vi "createInboundChannel.vi"(8 "error in (no error)":errorcluster, 11 "Connection.TCP in":refnum<class "Connection.TCP.lvclass">) -> (0 "error out":errorcluster, 2 "Authorization":T1, 3 "Connection.TCP out":refnum<class "Connection.TCP.lvclass">)   [LabVIEW 2013, in "Connection.TCP_GOSPL.lvlib" / "Connection.TCP.lvclass"]
uses:
  Connection.TCP.lvclass
  Connection/auth -- cluster.ctl
  Connection/Connection.lvclass
  Connection/Connection.lvclass/Connection.ctl
  Connection.TCP.lvclass/Connection.TCP.ctl
  <vilib>/LabVIEW Open Source Project/OpenURI/openURI.lvlib
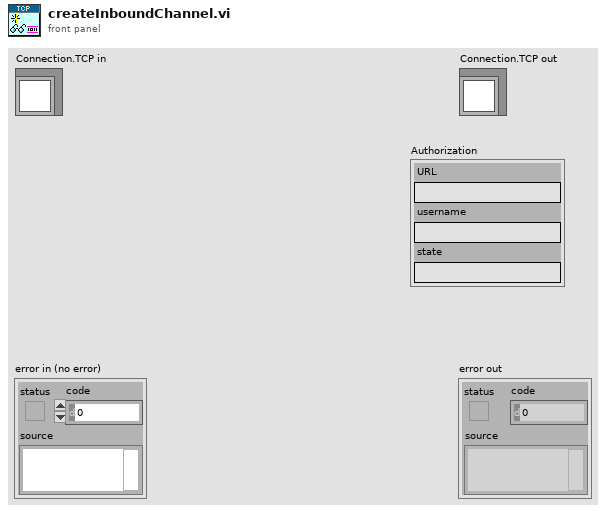
[diagram p1: front panel]
types:
  T1 = typedef "Connection_GOSPL.lvlib/Connection.lvclass/auth -- cluster.ctl" = cluster{"URL":string, "username":string, "state":string}
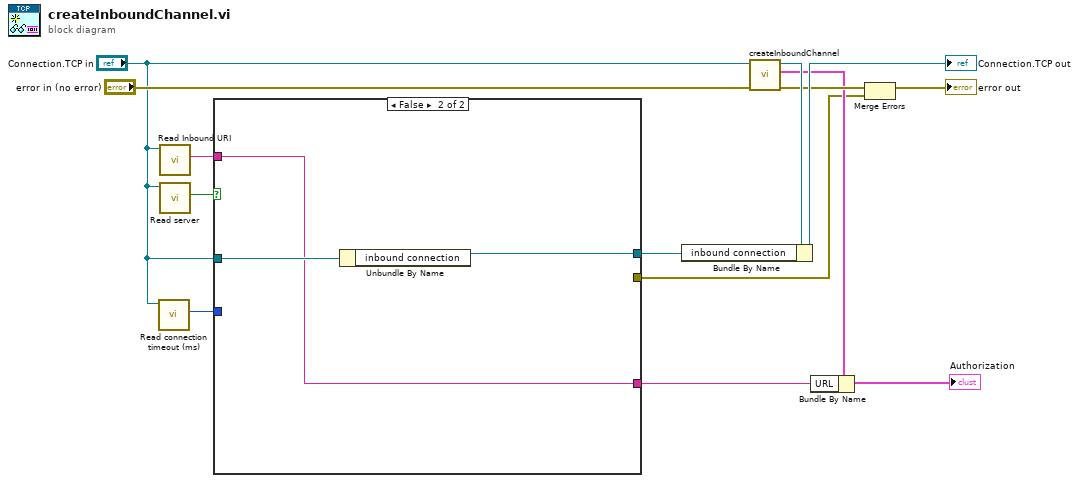
[diagram p0: block diagram]
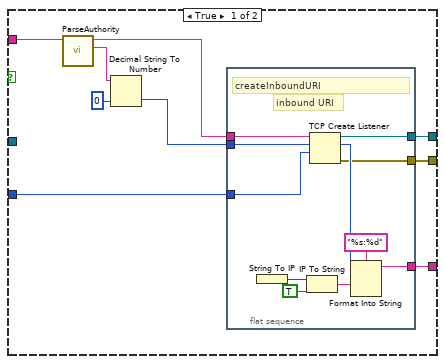
[diagram p2: hidden frame]
diagram:
  n1 = call "Read connection timeout (ms).vi"("Connection in"="Connection.TCP in") -> ("connection timeout (ms)"=w6:i32)  [unwired: 8 in, 2 out]
  n2 = call "Read Inbound URI.vi"("Connection in"="Connection.TCP in") -> ("Inbound URI"=w9:string)  [unwired: 9 in, 1 out]
  n3 = call "Read server.vi"("Connection in"="Connection.TCP in") -> ("server"=w2:bool)  [unwired: 9 in, 1 out]
  n4 = case shown="False" w2 {
    tunnel: w9 -> [w23 w35]
    tunnel: [w22 w35] -> w7
    tunnel: w6 -> [w20 _]
    tunnel: [w19 w36] -> w4
    tunnel: [w18 _] -> w3
    tunnel: "Connection.TCP in" -> [_ w37]
    frame True {
      n5 = call <vilib>:"ParseAuthority.vi"("authority"=w23) -> ("port"=w15:string, "host"=w21:string)  [unwired: 7 in, 2 out]
      n6 = Decimal String To Number(string=w15, default (0L)=u16 0 ("port")) -> (number=w17:u16)  [unwired: 1 in, 1 out]
      n7 = flat-sequence {
        tunnel: w21 -> [w34]
        tunnel: [w33] -> w19
        tunnel: [w27] -> w22
        tunnel: [w26] -> w18
        tunnel: w20 -> [w25]
        tunnel: w17 -> [w24]
        frame #0 {
          # "inbound URI"
          # "createInboundURI"
          n8 = String To IP() -> (0:w32:u32)  [unwired: 1 in]
          n9 = IP To String(1:TRUE ("dot notation? (F)"), 2:w32) -> (0:w30:string)
          n10 = TCP Create Listener(9:w25, 10:w24, 11:w34) -> (0:w26:errorcluster, 2:w28:u16, 3:w33:refnum<k5>)  [unwired: 2 in]
          n11 = Format Into String(format string="%s:%d", w30, w28) -> (resulting string=w27:string)  [unwired: 2 in, 1 out]
        }
      }
    }
    frame False {
      n12 = Unbundle By Name(w37) -> ("inbound connection"=w36:refnum<k5>)
    }
  }
  n13 = call-parent "createInboundChannel.vi"("error in (no error)"="error in (no error)", "Connection in"="Connection.TCP in") -> ("error out"=w11:errorcluster, "Authorization"=w8:T1, "Connection out"=w13:refnum<class "Connection.TCP.lvclass">)  [unwired: 7 in]
  n14 = Bundle By Name(cluster=w13, "inbound connection"=w4) -> (→"Connection.TCP out":refnum<class "Connection.TCP.lvclass">)
  n15 = Bundle By Name(cluster=w8, "URL"=w7) -> (→"Authorization":T1)
  n16 = Merge Errors(w11, w3) -> (→"error out":errorcluster)
